vi "Lab4Q6.vi"() -> ()   [LabVIEW 2021]
panel:
  out "Color Ball 5":string
  out "Y Ball 5":dbl
  out "X Ball 5":dbl
  out "Color Ball 4":string
  out "Y Ball 4":dbl
  out "X Ball 4":dbl
  out "Color Ball 3":string
  out "Y Ball 3":dbl
  out "X Ball 3":dbl
  out "Color Ball 2":string
  out "Y Ball 2":dbl
  out "X Ball 2":dbl
  out "Color Ball 1":string
  out "Y Ball 1":dbl
  out "X Ball 1":dbl
  out "2D Picture":picture
  in  "Size of Rectangle":i16=10
  in  "Display History":bool=TRUE
  out "purple_y":dbl
  out "purple_x":dbl
  out "orange_y":dbl
  out "newobstacle_y":dbl
  out "newobstacle_x":dbl
  out "orange_x":dbl
  out "Y":dbl
  out "X":dbl
  in  "SendValue 8":dbl
  in  "SendValue 7":dbl
  in  "SendValue 6":dbl
  in  "SendValue 5":dbl
  in  "SendValue 4":dbl
  in  "SendValue 3":dbl
  in  "SendValue 2":dbl
  in  "SendValue1":dbl
  in  "Send Button":bool
  in  "stop":bool
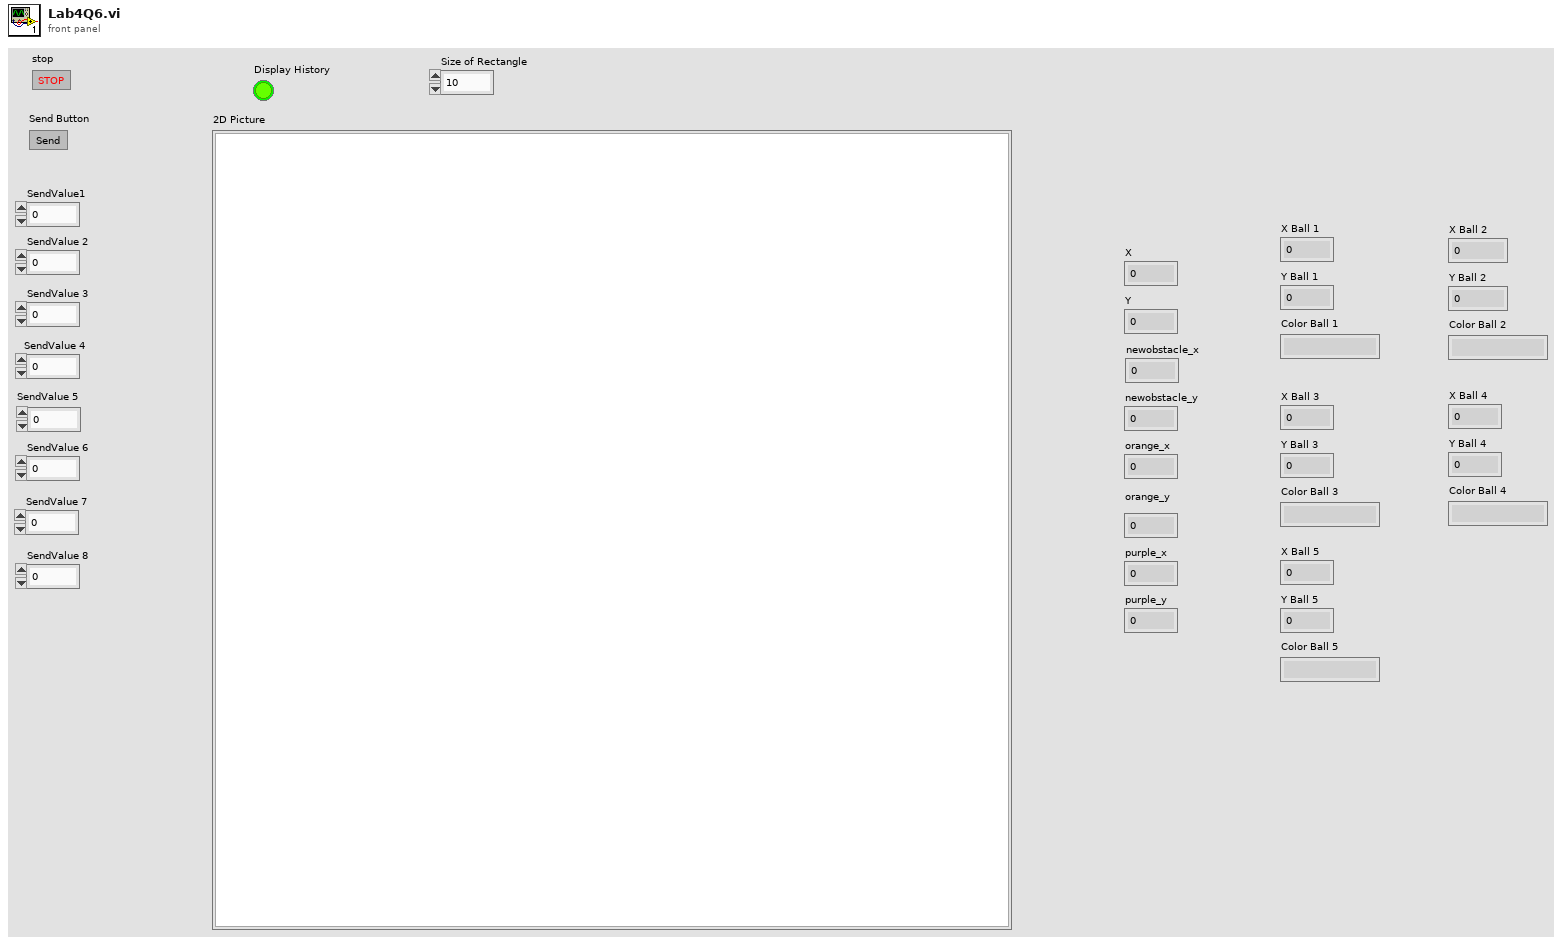
[diagram p1: front panel]
types:
  T1 = enum16{"Standard", "Buffered", "CRLF", "Immediate"}
  T2 = cluster{"Width":u16, "Style":enum32{"Solid", "Dash", "Dot", "DashDot", "DashDotDot"}}
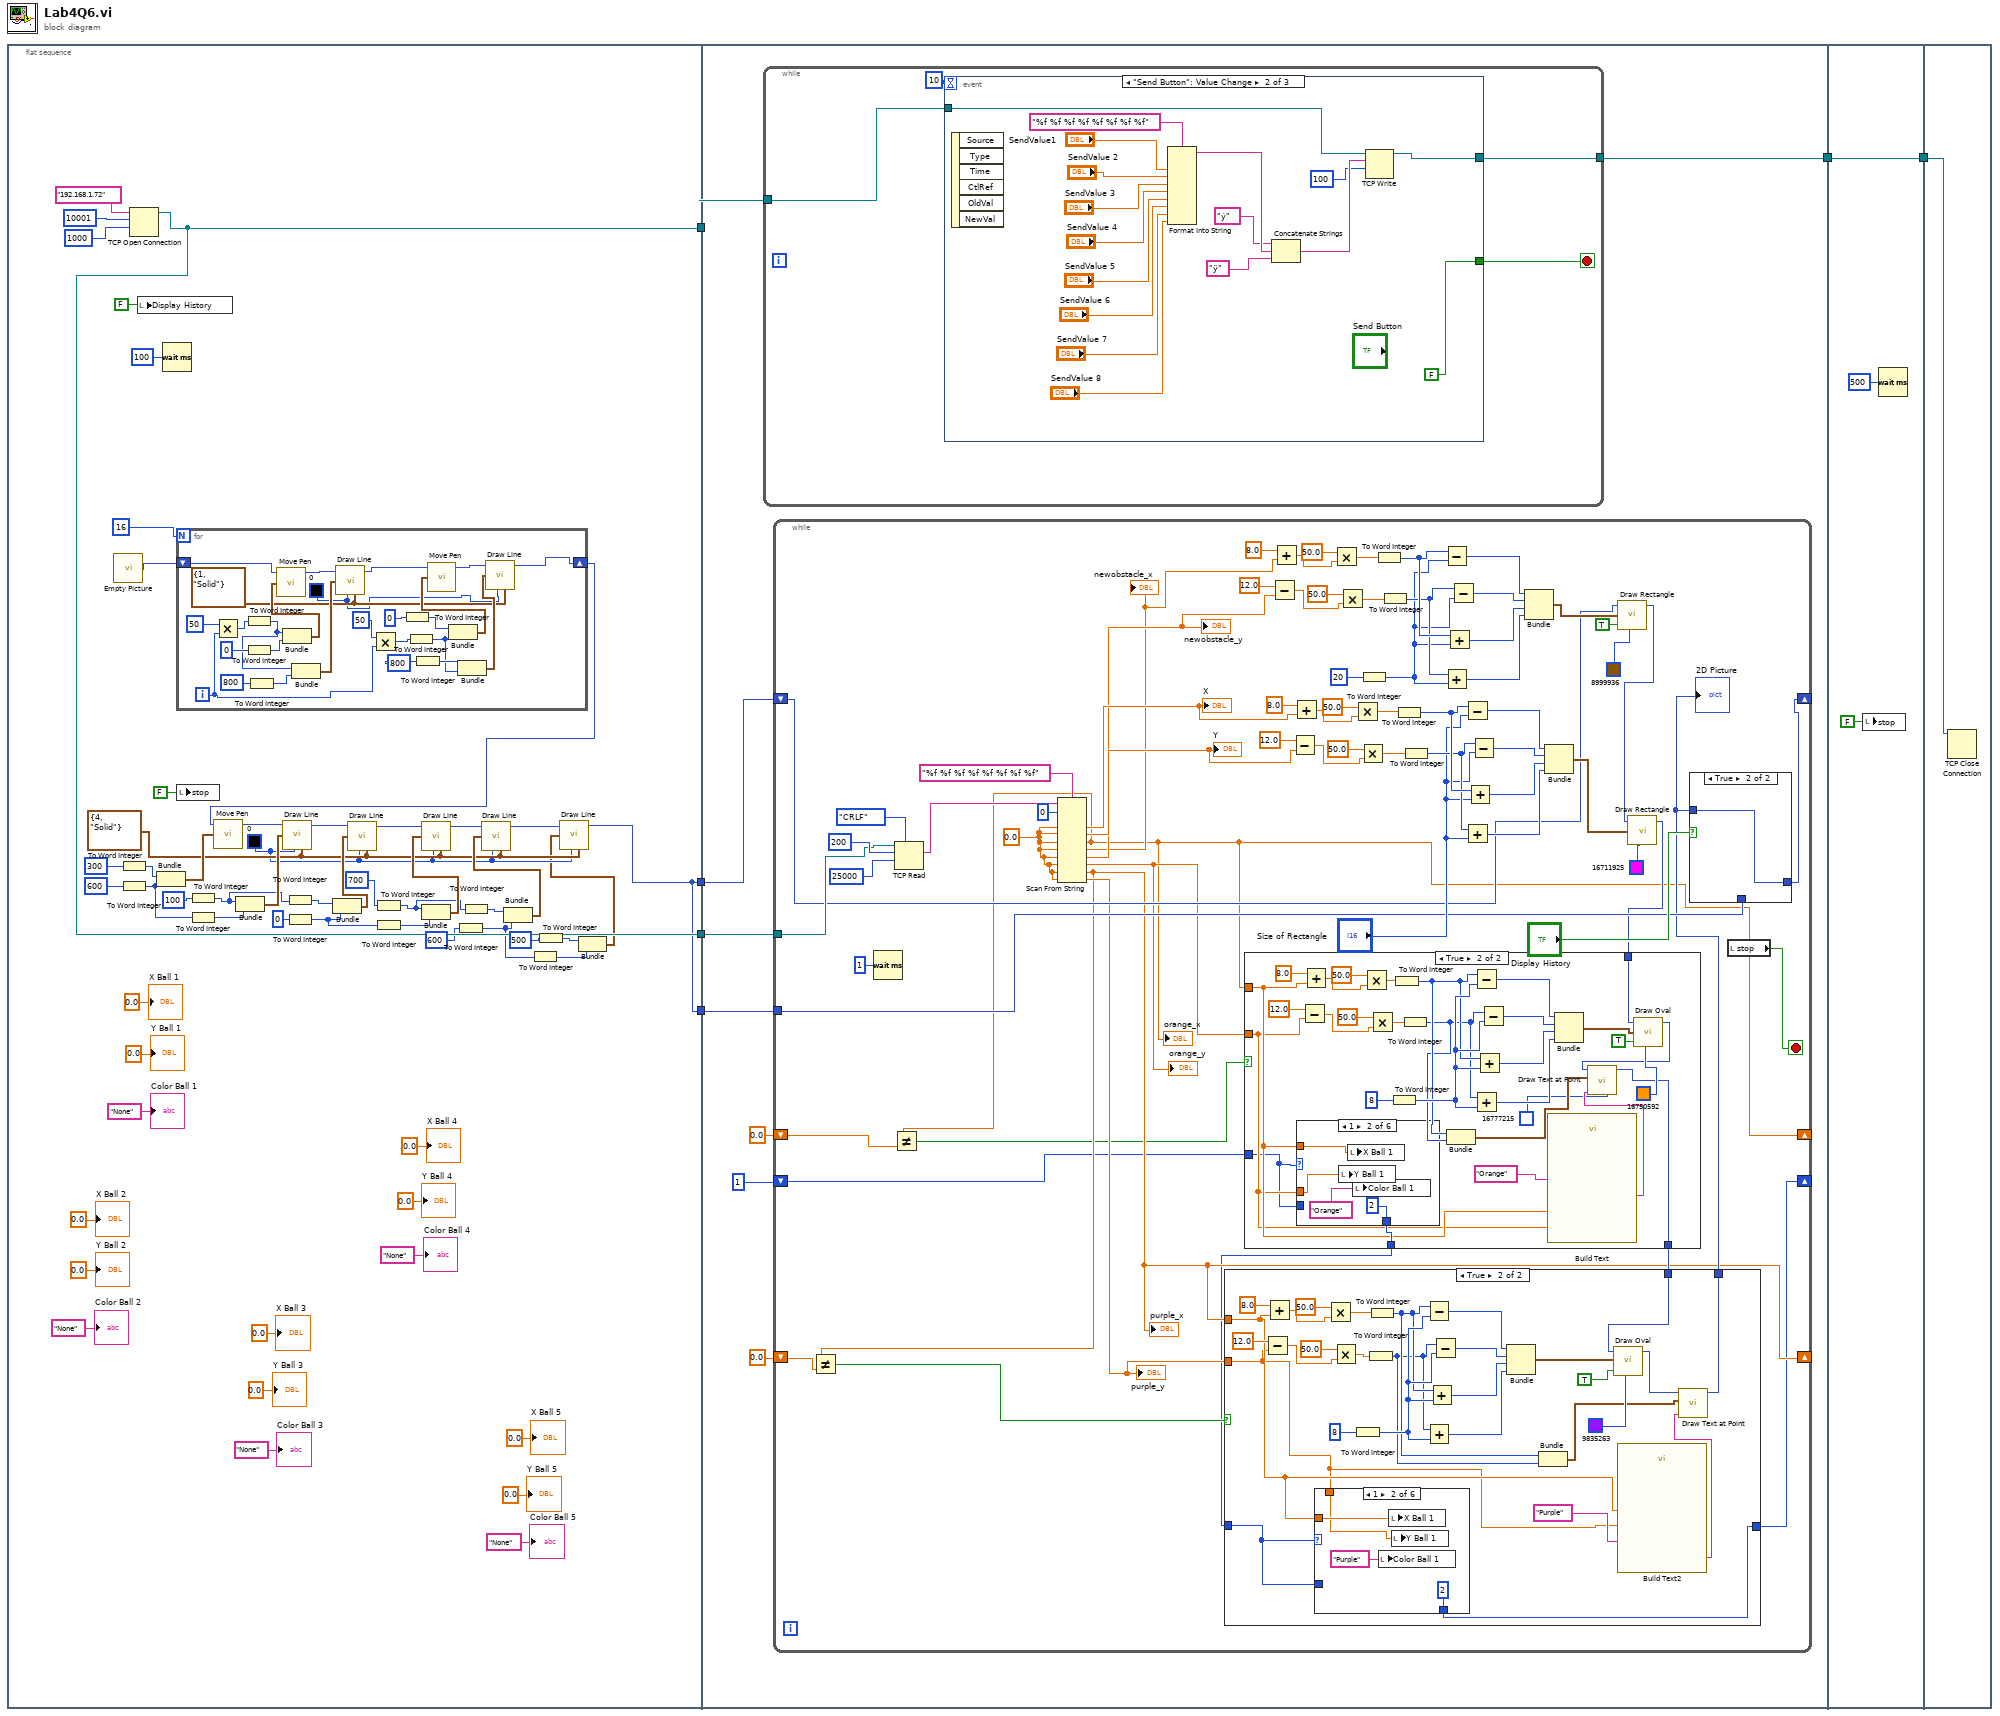
[diagram p0: block diagram]
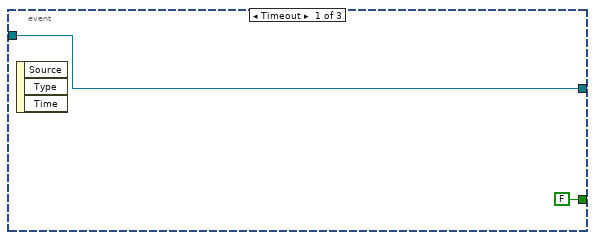
[diagram p2: hidden frame]
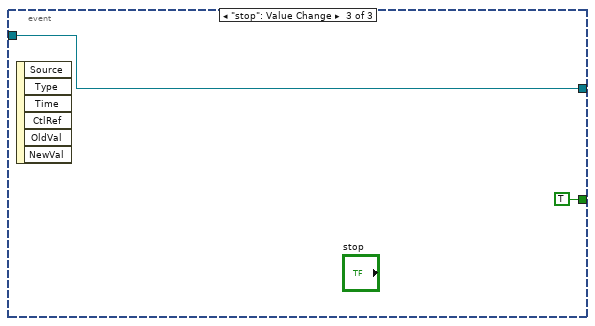
[diagram p3: hidden frame]
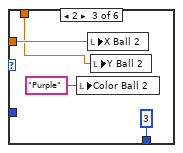
[diagram p6: hidden frame]
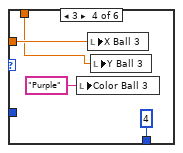
[diagram p7: hidden frame]
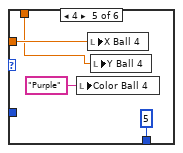
[diagram p8: hidden frame]
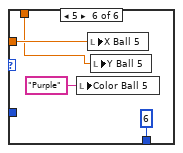
[diagram p9: hidden frame]
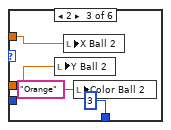
[diagram p12: hidden frame]
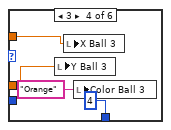
[diagram p13: hidden frame]
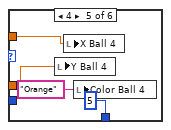
[diagram p14: hidden frame]
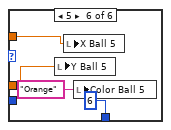
[diagram p15: hidden frame]
diagram:
  n1 = flat-sequence {
    tunnel: [w58] -> w6
    tunnel: [w58] -> w5
    tunnel: [w23] -> w2
    tunnel: [w23] -> w1
    tunnel: w6 -> [w98]
    tunnel: w5 -> [w96]
    tunnel: [w97] -> w3
    tunnel: w2 -> [w94]
    tunnel: w1 -> [w95]
    tunnel: [w302] -> w4
    tunnel: w3 -> [w302]
    tunnel: w4 -> [w303]
    frame #0 {
      w27 = u32 0 ("color(black)")
      w28 = T2 {"Width"=4, "Style"=enum."Solid"} ("pen")
      n2 = call "Empty Picture"() -> ("empty picture"=w56:picture)
      n3 = To Word Integer(number=i16 300) -> (16bit integer=w54:i16)
      n4 = To Word Integer(number=i16 600) -> (16bit integer=w48:i16)
      n5 = TCP Open Connection(address="192.168.1.72", remote port or service name=u16 10001, timeout ms (60000)=1000) -> (connection ID=w58:refnum<k5>)  [unwired: 2 in, 1 out]
      n6 = local write "Display History"(FALSE ("Display History")) -> ()
      n7 = Bundle(w54, w48) -> (w55:cluster{i16, i16})  [unwired: 1 in]
      n8 = Wait (ms)(milliseconds to wait=u32 100) -> ()  [unwired: 1 out]
      n9 = for {
        N: 16 -> [_]
        shift-right: [w65] -> w22
        shift-left: w56 -> [w66]
        i -> [w74]
        w67 = u32 0 ("color(black)")
        w68 = T2 {"Width"=1, "Style"=enum."Solid"} ("pen")
        n10 = Multiply(x=50, y=w74) -> (x*y=w87:i32)
        n11 = To Word Integer(number=w87) -> (16bit integer=w82:i16)
        n12 = To Word Integer(number=i16 0) -> (16bit integer=w85:i16)
        n13 = To Word Integer(number=i16 800) -> (16bit integer=w81:i16)
        n14 = Bundle(w82, w85) -> (w84:cluster{i16, i16})  [unwired: 1 in]
        n15 = call <vilib>:"Move Pen.vi"("new position"=w84, "picture"=w66) -> ("new picture"=w89:picture)  [unwired: 3 in]
        n16 = Bundle(w82, w81) -> (w79:cluster{i16, i16})  [unwired: 1 in]
        n17 = call <vilib>:"Draw Line.vi"("picture"=w89, "end point"=w79, "color(black)"=w67, "pen"=w68) -> ("new picture"=w88:picture)  [unwired: 5 in]
        n18 = Multiply(x=50, y=w74) -> (x*y=w78:i32)
        n19 = To Word Integer(number=i16 0) -> (16bit integer=w72:i16)
        n20 = To Word Integer(number=w78) -> (16bit integer=w71:i16)
        n21 = To Word Integer(number=i16 800) -> (16bit integer=w73:i16)
        n22 = Bundle(w72, w71) -> (w70:cluster{i16, i16})  [unwired: 1 in]
        n23 = call <vilib>:"Move Pen.vi"("new position"=w70, "picture"=w88) -> ("new picture"=w90:picture)  [unwired: 3 in]
        n24 = Bundle(w73, w71) -> (w69:cluster{i16, i16})  [unwired: 1 in]
        n25 = call <vilib>:"Draw Line.vi"("picture"=w90, "end point"=w69, "color(black)"=w67, "pen"=w68) -> ("new picture"=w65:picture)  [unwired: 5 in]
      }
      n26 = local write "stop"(FALSE ("stop")) -> ()
      n27 = To Word Integer(number=i16 100) -> (16bit integer=w44:i16)
      n28 = To Word Integer(number=w48) -> (16bit integer=w50:i16)
      n29 = call <vilib>:"Move Pen.vi"("new position"=w55, "picture"=w22) -> ("new picture"=w53:picture)  [unwired: 3 in]
      n30 = Bundle(w44, w50) -> (w49:cluster{i16, i16})  [unwired: 1 in]
      n31 = call <vilib>:"Draw Line.vi"("picture"=w53, "end point"=w49, "color(black)"=w27, "pen"=w28) -> ("new picture"=w46:picture)  [unwired: 5 in]
      n32 = To Word Integer(number=w44) -> (16bit integer=w45:i16)
      n33 = To Word Integer(number=i16 0) -> (16bit integer=w39:i16)
      n34 = Bundle(w45, w39) -> (w42:cluster{i16, i16})  [unwired: 1 in]
      n35 = call <vilib>:"Draw Line.vi"("picture"=w46, "end point"=w42, "color(black)"=w27, "pen"=w28) -> ("new picture"=w37:picture)  [unwired: 5 in]
      n36 = To Word Integer(number=i16 700) -> (16bit integer=w34:i16)
      n37 = To Word Integer(number=w39) -> (16bit integer=w41:i16)
      n38 = Bundle(w34, w41) -> (w38:cluster{i16, i16})  [unwired: 1 in]
      n39 = call <vilib>:"Draw Line.vi"("picture"=w37, "end point"=w38, "color(black)"=w27, "pen"=w28) -> ("new picture"=w36:picture)  [unwired: 5 in]
      n40 = To Word Integer(number=i16 600) -> (16bit integer=w24:i16)
      n41 = To Word Integer(number=w34) -> (16bit integer=w35:i16)
      n42 = Bundle(w35, w24) -> (w32:cluster{i16, i16})  [unwired: 1 in]
      n43 = call <vilib>:"Draw Line.vi"("picture"=w36, "end point"=w32, "color(black)"=w27, "pen"=w28) -> ("new picture"=w31:picture)  [unwired: 5 in]
      n44 = To Word Integer(number=w24) -> (16bit integer=w30:i16)
      n45 = To Word Integer(number=i16 500) -> (16bit integer=w29:i16)
      n46 = Bundle(w29, w30) -> (w26:cluster{i16, i16})  [unwired: 1 in]
      n47 = call <vilib>:"Draw Line.vi"("picture"=w31, "end point"=w26, "color(black)"=w27, "pen"=w28) -> ("new picture"=w23:picture)  [unwired: 5 in]
      "X Ball 1" <- 0.0 ("Ball1X")
      "Y Ball 1" <- 0.0 ("Ball1Y")
      "Color Ball 1" <- "None" ("Ball 1 Color")
      "Color Ball 2" <- "None" ("Color Ball 2")
      "Color Ball 3" <- "None" ("Color Ball 3")
      "X Ball 5" <- 0.0 ("X Ball 5")
      "Y Ball 5" <- 0.0 ("Y Ball 5")
      "Color Ball 5" <- "None" ("Color Ball 5")
      "X Ball 3" <- 0.0 ("X Ball 3")
      "Y Ball 3" <- 0.0 ("Y Ball 3")
      "Color Ball 4" <- "None" ("Color Ball 4")
      "X Ball 2" <- 0.0 ("X Ball 2")
      "Y Ball 2" <- 0.0 ("Y Ball 2")
      "X Ball 4" <- 0.0 ("X Ball 4")
      "Y Ball 4" <- 0.0 ("Y Ball 4")
    }
    frame #1 {
      n48 = while {
        tunnel: w98 -> [w101]
        tunnel: [w99] -> w97
        stop <- w100 stop-if-true
        n49 = event shown="[1] \"Send Button\": Value Change" {
          selector: _ -> [_ _ _]
          dyn-events: _ -> [_ _ _]
          timeout: 10 -> [_ _ _]
          tunnel: w101 -> [w103 w107 w122]
          tunnel: [FALSE FALSE TRUE] -> w100
          tunnel: [w103 w105 w122] -> w99
          event Timeout {
            n50 = event-data() -> ()  [unwired: 1 in, 3 out]
          }
          event "Send Button": Value Change {
            n51 = event-data() -> ()  [unwired: 1 in, 6 out]
            n52 = Format Into String(format string="%f %f %f %f %f %f %f %f", "SendValue1", "SendValue 2", "SendValue 3", "SendValue 4", "SendValue 5", "SendValue 6", "SendValue 7", "SendValue 8") -> (resulting string=w112:string)  [unwired: 2 in, 1 out]
            n53 = Concatenate Strings("ý" ("string"), w112, "ÿ" ("string")) -> (w109:string)
            n54 = TCP Write(connection ID=w107, data in=w109, 9:100 ("timeout ms (25000)")) -> (connection ID out=w105:refnum<k5>)  [unwired: 1 in, 2 out]
          }
          event "stop": Value Change {
            n55 = event-data() -> ()  [unwired: 1 in, 6 out]
          }
        }
      }
      n56 = while {
        shift-right: [w161] -> _
        shift-left: w94 -> [w140]
        tunnel: w96 -> [w187]
        tunnel: w95 -> [w162]
        shift-right: [w131] -> _
        shift-left: 0.0 ("default value 1") -> [w132]
        shift-right: [w129] -> _
        shift-left: 0.0 ("default value 1") -> [w130]
        shift-right: [w124] -> _
        shift-left: 1 -> [w127]
        stop <- w164 stop-if-true
        w183 = 0.0 ("default value 1")
        n57 = Wait (ms)(milliseconds to wait=u32 1) -> ()  [unwired: 1 out]
        n58 = TCP Read(connection ID=w187, bytes to read=200, 7:T1."CRLF" ("mode (standard)"), 9:25000 ("timeout ms (25000)")) -> (data out=w185:string)  [unwired: 1 in, 2 out]
        n59 = Scan From String(format string="%f %f %f %f %f %f %f %f", input string=w185, initial scan location=u32 0, default 1=w183, default 2=w183, default 3=w183, default 4=w183, default 5=w183, default 6=w183, default 7=w183, default 8=w183) -> (output 1=w180:dbl, output 2=w178:dbl, output 3=w131:dbl, output 4=w142:dbl, output 5=w143:dbl, output 6=w136:dbl, output 7=w129:dbl, output 8=w135:dbl)  [unwired: 1 in, 3 out]
        "X" <- w180
        "Y" <- w178
        "orange_x" <- w131
        "newobstacle_x" <- w142
        "newobstacle_y" <- w143
        "orange_y" <- w136
        "purple_x" <- w129
        "purple_y" <- w135
        n60 = Not Equal?(x=w129, y=w130) -> (x != y?=w126:bool)
        n61 = Not Equal?(x=w131, y=w132) -> (x != y?=w128:bool)
        n62 = Subtract(x=12.0, y=w143) -> (x-y=w154:dbl)
        n63 = Add(x=8.0, y=w142) -> (x+y=w155:dbl)
        n64 = Subtract(x=12.0, y=w178) -> (x-y=w174:dbl)
        n65 = Add(x=8.0, y=w180) -> (x+y=w175:dbl)
        n66 = Multiply(x=50.0, y=w155) -> (x*y=w153:dbl)
        n67 = Multiply(x=50.0, y=w154) -> (x*y=w152:dbl)
        n68 = Multiply(x=50.0, y=w175) -> (x*y=w173:dbl)
        n69 = Multiply(x=50.0, y=w174) -> (x*y=w172:dbl)
        n70 = To Word Integer(number=i16 20) -> (16bit integer=w145:i16)
        n71 = To Word Integer(number=w153) -> (16bit integer=w151:i16)
        n72 = To Word Integer(number=w152) -> (16bit integer=w150:i16)
        n73 = To Word Integer(number=w173) -> (16bit integer=w171:i16)
        n74 = To Word Integer(number=w172) -> (16bit integer=w170:i16)
        n75 = Subtract(x=w151, y=w145) -> (x-y=w149:i16)
        n76 = Add(x=w150, y=w145) -> (x+y=w146:i16)
        n77 = Add(x=w151, y=w145) -> (x+y=w147:i16)
        n78 = Subtract(x=w150, y=w145) -> (x-y=w148:i16)
        n79 = Subtract(x=w171, y="Size of Rectangle") -> (x-y=w168:i16)
        n80 = Add(x=w170, y="Size of Rectangle") -> (x+y=w165:i16)
        n81 = Add(x=w171, y="Size of Rectangle") -> (x+y=w166:i16)
        n82 = Subtract(x=w170, y="Size of Rectangle") -> (x-y=w167:i16)
        n83 = Bundle(w149, w148, w147, w146) -> (w141:cluster{i16, i16, i16, i16})  [unwired: 1 in]
        n84 = Bundle(w168, w167, w166, w165) -> (w192:cluster{i16, i16, i16, i16})  [unwired: 1 in]
        n85 = call <vilib>:"Draw Rectangle.vi"("picture"=w140, "rect"=w141, "fill?(F)"=TRUE, "color(black)"=u32 8999936) -> ("new picture"=w139:picture)  [unwired: 5 in]
        n86 = call <vilib>:"Draw Rectangle.vi"("picture"=w139, "rect"=w192, "color(black)"=u32 16711925) -> ("new picture"=w137:picture)  [unwired: 6 in]
        n87 = case shown="True" w128 {
          tunnel: w137 -> [w246 w259]
          tunnel: w136 -> [_ w249]
          tunnel: [w246 w255] -> w134
          tunnel: w131 -> [_ w250]
          tunnel: w127 -> [w245 w247]
          tunnel: [w245 w251] -> w125
          frame False {
          }
          frame True {
            n88 = case shown="1" w247 {
              tunnel: [w277 2 3 4 5 6] -> w251
              tunnel: w247 -> [w277 _ _ _ _ _]
              tunnel: w250 -> [_ w280 w284 w288 w292 w296]
              tunnel: w249 -> [_ w279 w283 w287 w291 w295]
              frame 0, Default {
              }
              frame 1 {
                n89 = local write "Y Ball 1"(w279) -> ()
                n90 = local write "X Ball 1"(w280) -> ()
                n91 = local write "Color Ball 1"("Orange" ("Ball 1 Color")) -> ()
              }
              frame 2 {
                n92 = local write "Y Ball 2"(w283) -> ()
                n93 = local write "X Ball 2"(w284) -> ()
                n94 = local write "Color Ball 2"("Orange" ("Ball 1 Color")) -> ()
              }
              frame 3 {
                n95 = local write "Y Ball 3"(w287) -> ()
                n96 = local write "X Ball 3"(w288) -> ()
                n97 = local write "Color Ball 3"("Orange" ("Ball 1 Color")) -> ()
              }
              frame 4 {
                n98 = local write "Y Ball 4"(w291) -> ()
                n99 = local write "X Ball 4"(w292) -> ()
                n100 = local write "Color Ball 4"("Orange" ("Ball 1 Color")) -> ()
              }
              frame 5 {
                n101 = local write "Y Ball 5"(w295) -> ()
                n102 = local write "X Ball 5"(w296) -> ()
                n103 = local write "Color Ball 5"("Orange" ("Ball 1 Color")) -> ()
              }
            }
            n104 = Subtract(x=12.0, y=w249) -> (x-y=w271:dbl)
            n105 = Add(x=8.0, y=w250) -> (x+y=w272:dbl)
            n106 = Multiply(x=50.0, y=w272) -> (x*y=w270:dbl)
            n107 = Multiply(x=50.0, y=w271) -> (x*y=w269:dbl)
            n108 = To Word Integer(number=i16 8) -> (16bit integer=w264:i16)
            n109 = To Word Integer(number=w270) -> (16bit integer=w254:i16)
            n110 = To Word Integer(number=w269) -> (16bit integer=w253:i16)
            n111 = Bundle(w254, w253) -> (w252:cluster{i16, i16})  [unwired: 1 in]
            n112 = Subtract(x=w254, y=w264) -> (x-y=w268:i16)
            n113 = Add(x=w253, y=w264) -> (x+y=w265:i16)
            n114 = Add(x=w254, y=w264) -> (x+y=w266:i16)
            n115 = Subtract(x=w253, y=w264) -> (x-y=w267:i16)
            n116 = call "Build Text"("xcoord"=w250, "ycoord"=w249, "color"="Orange") -> ("Result"=w258:string)  [unwired: 11 in, 1 out]
            n117 = Bundle(w268, w267, w266, w265) -> (w260:cluster{i16, i16, i16, i16})  [unwired: 1 in]
            n118 = call <vilib>:"Draw Oval.vi"("picture"=w259, "rect"=w260, "fill?(F)"=TRUE, "color(black)"=u32 16750592) -> ("new picture"=w256:picture)  [unwired: 5 in]
            n119 = call <vilib>:"Draw Text at Point.vi"("BG color(transparent)"=u32 16777215, "text"=w258, "origin"=w252, "picture"=w256) -> ("new picture"=w255:picture)  [unwired: 6 in, 1 out]
          }
        }
        n120 = case shown="True" w126 {
          tunnel: w135 -> [_ w197]
          tunnel: w134 -> [w194 w205]
          tunnel: [w194 w203] -> w133
          tunnel: w129 -> [_ w198]
          tunnel: w125 -> [w193 w196]
          tunnel: [w193 w195] -> w124
          frame False {
          }
          frame True {
            n121 = Subtract(x=12.0, y=w197) -> (x-y=w218:dbl)
            n122 = Add(x=8.0, y=w198) -> (x+y=w219:dbl)
            n123 = case shown="1" w196 {
              tunnel: w198 -> [_ w227 w231 w235 w239 w243]
              tunnel: w197 -> [_ w226 w230 w234 w238 w242]
              tunnel: w196 -> [w224 _ _ _ _ _]
              tunnel: [w224 2 3 4 5 6] -> w195
              frame 0, Default {
              }
              frame 1 {
                n124 = local write "Color Ball 1"("Purple" ("Color Ball 1")) -> ()
                n125 = local write "X Ball 1"(w227) -> ()
                n126 = local write "Y Ball 1"(w226) -> ()
              }
              frame 2 {
                n127 = local write "Color Ball 2"("Purple" ("Color Ball 1")) -> ()
                n128 = local write "X Ball 2"(w231) -> ()
                n129 = local write "Y Ball 2"(w230) -> ()
              }
              frame 3 {
                n130 = local write "Color Ball 3"("Purple" ("Color Ball 1")) -> ()
                n131 = local write "X Ball 3"(w235) -> ()
                n132 = local write "Y Ball 3"(w234) -> ()
              }
              frame 4 {
                n133 = local write "Color Ball 4"("Purple" ("Color Ball 1")) -> ()
                n134 = local write "X Ball 4"(w239) -> ()
                n135 = local write "Y Ball 4"(w238) -> ()
              }
              frame 5 {
                n136 = local write "Color Ball 5"("Purple" ("Color Ball 1")) -> ()
                n137 = local write "X Ball 5"(w243) -> ()
                n138 = local write "Y Ball 5"(w242) -> ()
              }
            }
            n139 = Multiply(x=50.0, y=w219) -> (x*y=w217:dbl)
            n140 = Multiply(x=50.0, y=w218) -> (x*y=w216:dbl)
            n141 = To Word Integer(number=i16 8) -> (16bit integer=w211:i16)
            n142 = To Word Integer(number=w216) -> (16bit integer=w200:i16)
            n143 = To Word Integer(number=w217) -> (16bit integer=w201:i16)
            n144 = Subtract(x=w201, y=w211) -> (x-y=w215:i16)
            n145 = Add(x=w200, y=w211) -> (x+y=w212:i16)
            n146 = Add(x=w201, y=w211) -> (x+y=w213:i16)
            n147 = Subtract(x=w200, y=w211) -> (x-y=w214:i16)
            n148 = Bundle(w215, w214, w213, w212) -> (w209:cluster{i16, i16, i16, i16})  [unwired: 1 in]
            n149 = Bundle(w201, w200) -> (w199:cluster{i16, i16})  [unwired: 1 in]
            n150 = call <vilib>:"Draw Oval.vi"("picture"=w205, "rect"=w209, "fill?(F)"=TRUE, "color(black)"=u32 9835263) -> ("new picture"=w204:picture)  [unwired: 5 in]
            n151 = call "Build Text2"("xcoord"=w198, "ycoord"=w197, "color"="Purple") -> ("Result"=w202:string)  [unwired: 11 in, 1 out]
            n152 = call <vilib>:"Draw Text at Point.vi"("text"=w202, "origin"=w199, "picture"=w204) -> ("new picture"=w203:picture)  [unwired: 7 in, 1 out]
          }
        }
        "2D Picture" <- w133
        n153 = case shown="True" "Display History" {
          tunnel: [w298 w299] -> w161
          tunnel: w133 -> [_ w299]
          tunnel: w162 -> [w298 _]
          frame False {
          }
          frame True {
          }
        }
        n154 = local read "stop"() -> (w164:bool)
      }
    }
    frame #2 {
      n155 = local write "stop"(FALSE ("stop")) -> ()
      n156 = Wait (ms)(milliseconds to wait=u32 500) -> ()  [unwired: 1 out]
    }
    frame #3 {
      n157 = TCP Close Connection(connection ID=w303) -> ()  [unwired: 2 in, 2 out]
    }
  }
